vi "Overlay Targets Example.vi"(11 "Image":T1) -> (3 "Camera Image":T1(plugin-control))   [LabVIEW 2011]
uses:
  <vilib>/vision/Image Controls.llb/IMAQ Image.ctl
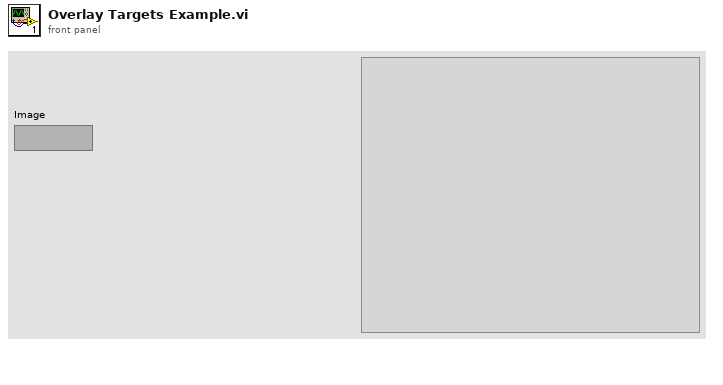
[diagram p1: front panel]
types:
  T1 = typedef "IMAQ Image.ctl" = refnum<image>
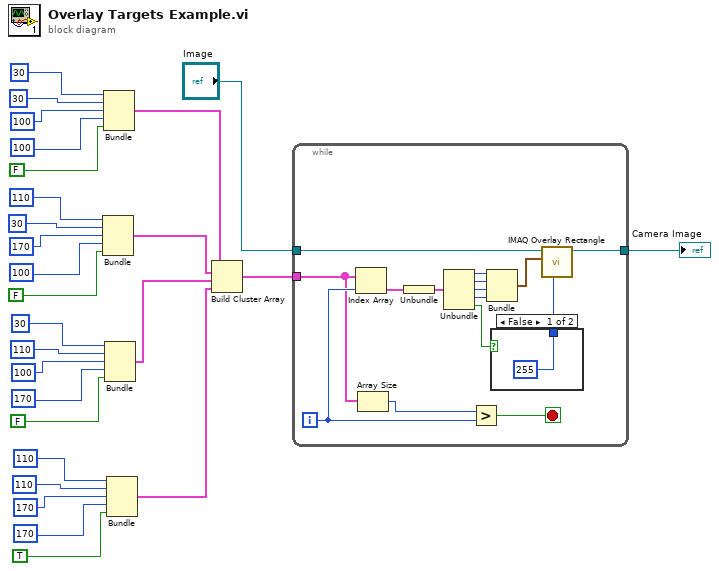
[diagram p0: block diagram]
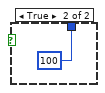
[diagram p2: hidden frame]
diagram:
  n1 = Bundle(110, 30, 170, 100, FALSE) -> (w5:cluster{i32, i32, i32, i32, bool})  [unwired: 1 in]
  n2 = Bundle(30, 30, 100, 100, FALSE) -> (w4:cluster{i32, i32, i32, i32, bool})  [unwired: 1 in]
  n3 = Bundle(30, 110, 100, 170, FALSE) -> (w6:cluster{i32, i32, i32, i32, bool})  [unwired: 1 in]
  n4 = Bundle(110, 110, 170, 170, TRUE) -> (w7:cluster{i32, i32, i32, i32, bool})  [unwired: 1 in]
  n5 = Build Cluster Array(w4, w5, w6, w7) -> (w3:cluster{cluster{i32, i32, i32, i32, bool}}[])
  n6 = while {
    tunnel: [w42] -> w2
    tunnel: w3 -> [w38]
    tunnel: "Image" -> [w28]
    i -> [w39]
    stop <- w40 stop-if-true
    n7 = Index Array(array=w38, index=w39) -> (element=w36:cluster{cluster{i32, i32, i32, i32, bool}})
    n8 = Array Size(array=w38) -> (size(s)=w41:i32)
    n9 = Unbundle(w36) -> (w37:cluster{i32, i32, i32, i32, bool})
    n10 = Unbundle(w37) -> (w35:i32, w34:i32, w33:i32, w32:i32, w30:bool)
    n11 = Greater?(x=w41, y=w39) -> (0:w40:bool)
    n12 = Bundle(w35, w34, w33, w32) -> (w31:cluster{i32, i32, i32, i32})  [unwired: 1 in]
    n13 = case shown="False" w30 {
      tunnel: [255 100] -> w29
      frame False {
      }
      frame True {
      }
    }
    n14 = call "IMAQ Overlay Rectangle"("Color"=w29, "Rectangle"=w31, "Image"=w28) -> ("Image Out"=w42:T1)  [unwired: 7 in, 1 out]
  }
  "Camera Image" <- w2
